vi "Type.vi"(11 "StringPanel in":refnum<class "StringPanel.lvclass">) -> (2 "Type":refnum<class "Type.lvclass">)   [LabVIEW 2020, in "Conditum-Tools.lvlib" / "StringPanel.lvclass"]
uses:
  StringPanel.lvclass
  Conditum/Columns/Type/Type.lvclass
  StringPanel.lvclass/StringPanel.ctl
  Conditum/Columns/String/String.lvclass
  C:/dev/lv20CE/lv-conditum/Conditum/Columns/Type/Type.lvclass
  C:/dev/lv20CE/lv-conditum/Conditum/Columns/String/String.lvclass
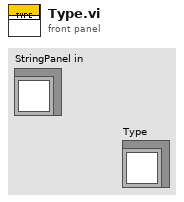
[diagram p1: front panel]
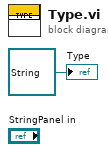
[diagram p0: block diagram]
diagram:
  "Type" <- refnum<class "String.lvclass"> refnum ("Conditum:Columns:String.lvclass")
